vi "lab4_4.vi"() -> ()   [LabVIEW 2021]
panel:
  in  "stop":bool
  out "Numeric":dbl
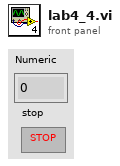
[diagram p1: front panel]
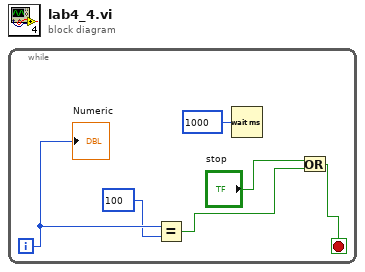
[diagram p0: block diagram]
diagram:
  n1 = while {
    i -> [w2]
    stop <- w4 stop-if-true
    n2 = Equal?(x=w2, y=100) -> (x = y?=w3:bool)
    n3 = Wait (ms)(milliseconds to wait=u32 1000) -> ()  [unwired: 1 out]
    n4 = Or(x="stop", y=w3) -> (x .or. y?=w4:bool)
    "Numeric" <- w2
  }
